vi "Split String.vi"(6 "Split Pattern":string, 10 "Input String":string) -> (2 "Split String":string[](array[string]))   [LabVIEW 2020, in "String Manipulation.lvlib"]
uses:
  <vilib>/gpm_packages/@cs/linked-list/Source/String Manipulation/String Manipulation.lvlib
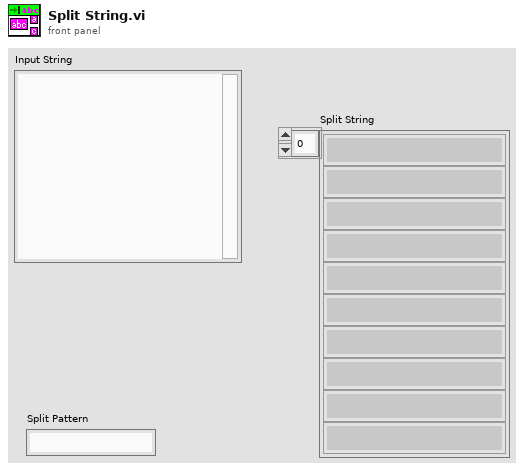
[diagram p1: front panel]
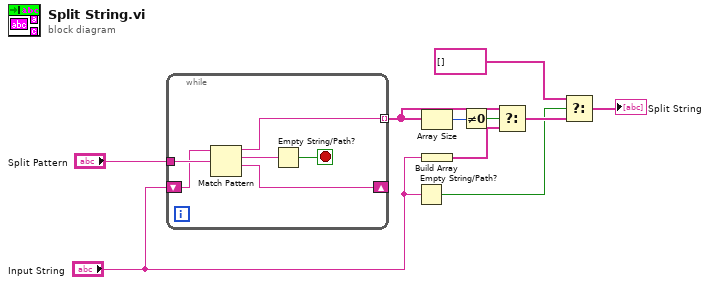
[diagram p0: block diagram]
diagram:
  n1 = while {
    tunnel: [w15] -> w7 mode=indexing
    shift-right: [w13] -> _
    shift-left: "Input String" -> [w11]
    tunnel: "Split Pattern" -> [w12]
    stop <- w16 stop-if-true
    n2 = Match Pattern(string=w11, regular expression=w12) -> (before substring=w15:string, match substring=w14:string, after substring=w13:string)  [unwired: 1 in, 1 out]
    n3 = Empty String/Path?(string/path=w14) -> (empty?=w16:bool)
  }
  n4 = Empty String/Path?(string/path="Input String") -> (empty?=w4:bool)
  n5 = Array Size(array=w7) -> (size(s)=w10:i32)
  n6 = Build Array("Input String") -> (w8:string[])
  n7 = Not Equal To 0?(x=w10) -> (x != 0?=w9:bool)
  n8 = Select(t=w7, s=w9, f=w8) -> (s? t:f=w5:string[])
  n9 = Select(t=string[] [], s=w4, f=w5) -> (s? t:f=→"Split String":string[])
